vi "Read Temperature DBL.vi"(8 "error in":errorcluster, 10 "Source":string, 11 "Virtual Thermometer in":refnum<class "Virtual Thermometer.lvclass">) -> (0 "error out":errorcluster, 1 "Time Stamp":timestamp format="%<%x %.3X>T", 2 "Temperature":dbl, 3 "Virtual Thermometer out":refnum<class "Virtual Thermometer.lvclass">)   [LabVIEW 2024, in "Virtual Thermometer.lvclass"]
uses:
  Virtual Thermometer.lvclass
  Virtual Thermometer.lvclass/Virtual Thermometer.ctl
  Interfaces/IRead Temperature/IRead Temperature.lvclass
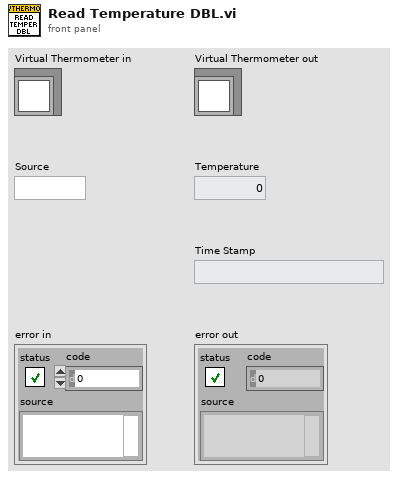
[diagram p1: front panel]
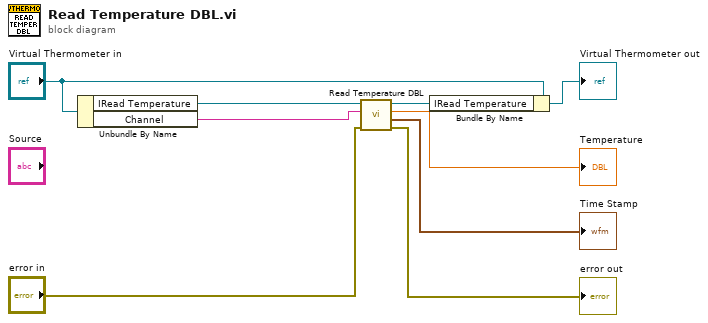
[diagram p0: block diagram]
diagram:
  n1 = Unbundle By Name("Virtual Thermometer in") -> ("IRead Temperature"=w9:refnum<class "IRead Temperature.lvclass">, "Channel"=w1:string)
  n2 = call-dynamic "Read Temperature DBL.vi"("error in"="error in", "Source"=w1, "IRead Temperature in"=w9) -> ("error out"=→"error out":errorcluster, "Time Stamp"=→"Time Stamp":timestamp, "Temperature"=→"Temperature":dbl, "IRead Temperature out"=w4:refnum<class "IRead Temperature.lvclass">)  [unwired: 5 in]
  n3 = Bundle By Name(cluster="Virtual Thermometer in", "IRead Temperature"=w4) -> (→"Virtual Thermometer out":refnum<class "Virtual Thermometer.lvclass">)
